vi "RSNRPZ Get Status Update Time.vi"(8 "error in (no error)":errorcluster, 10 "Channel (1)":i32=1, 11 "VISA session":refnum<visa-resource-name> caption="VISA resource name") -> (0 "error out":errorcluster, 2 "Status Update Time":dbl format="%^.3e", 3 "dup VISA session":refnum<visa-resource-name> caption="VISA resource name")   [LabVIEW 2010]
doc: "This VI gets status update time.\n\nNote:\n\n1) This VI is available only for NRP-Z81.\n\nRemote-control command(s):\nSYST:SUT"
uses:
  rsnrpz_32.dll
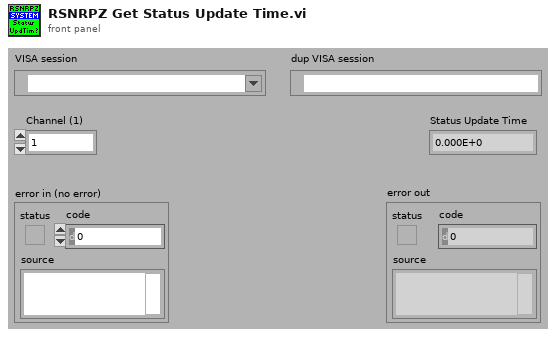
[diagram p1: front panel]
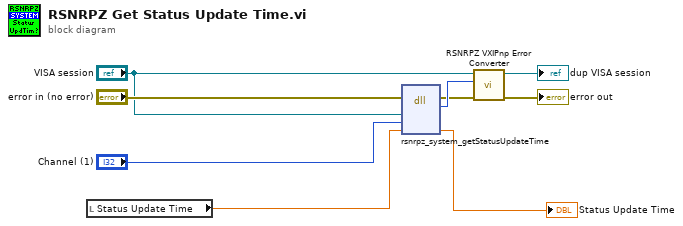
[diagram p0: block diagram]
diagram:
  n1 = local read "Status Update Time"() -> (w7:dbl)
  n2 = dll-call lib="rsnrpz_32.dll" fn="rsnrpz_system_getStatusUpdateTime"(error in="error in (no error)", "Instrument Handle"="VISA session", "Channel"="Channel (1)", "Status Update Time"=w7) -> (error out=w5:errorcluster, "Status"=w9:i32, "Status Update Time"=→"Status Update Time":dbl)  [unwired: 4 in, 1 out]
  n3 = call <instrlib>:"RSNRPZ VXIPnp Error Converter.vi"("error in"=w5, "VXIPnp error code"=w9, "VISA session"="VISA session") -> ("error out"=→"error out":errorcluster, "dup VISA session"=→"dup VISA session":refnum<visa-resource-name>)  [unwired: 7 in]
